vi "ShooterSpeedRegulateV4.1.vi"(8 "Reset PID":bool, 11 "Shooter Speed":T1(ring)) -> (2 "Voltage Output":dbl, 3 "GO GO GO":bool)   [LabVIEW 2012]
uses:
  Robot Global Data.vi
  Max'sToolKit/ConvertVoltageToPercentVbs.vi
panel:
  out "Motor Outputs":cluster{"Error":dbl, dbl, i32}(graph)
  out "Setpoint":dbl
  out "Error (RPS)":dbl
  out "Output":dbl
  out "Speed (RPS)":dbl
  # "Wheel Speed\n0 - DEFAULT/OFF\n1 - close 3pt\n2 - far 3pt\n3 - feeder shot\n4- upside down far 3pt\n\nno more at the moment"
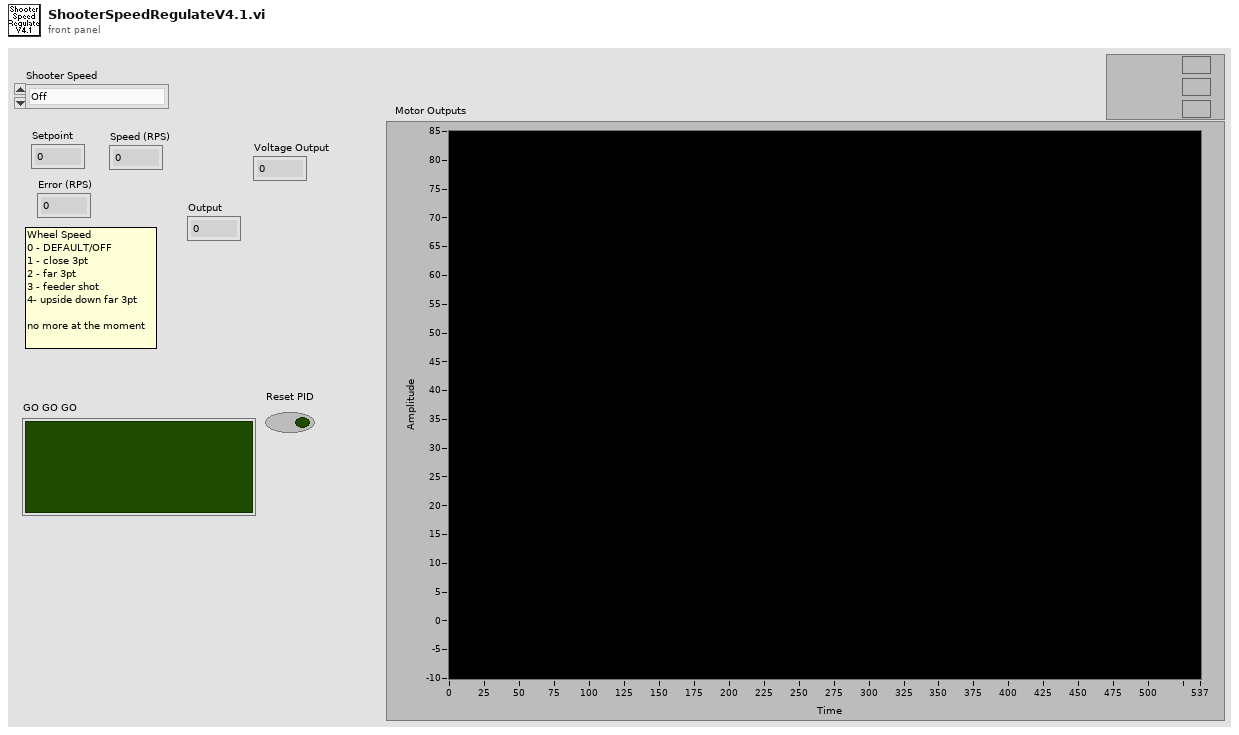
[diagram p1: front panel]
types:
  T1 = enum16{"Off", "Close Pyramid 3pt", "Far Pyramid 3pt", "Feeder Shot", "UD Far 3pt Shot"}
  T2 = cluster{"Target Voltage":dbl, "Target Speed":dbl, "Angle Up?":bool}[]
  T3 = cluster{"Target Voltage":dbl, "Target Speed":dbl, "Angle Up?":bool}
  T4 = typedef "WPI_EncoderDevRef.ctl" = cluster{"DevStatus":errorcluster, "EncoderIndex":T5, "CounterIndex":T6, "DistancePerCount":dbl, "Decoding Type":T7}
  T5 = typedef "FPGA_EncoderIdx.ctl" = enum8{"Enc 0", "Enc 1", "Enc 2", "Enc 3", "Invalid"}
  T6 = typedef "FPGA_CounterCtrSystemIndex.ctl" = enum8{"Ctr 0", "Ctr 1", "Ctr 2", "Ctr 3", "Ctr 4", "Ctr 5", "Ctr 6", "Ctr 7", "Invalid"}
  T7 = typedef "WPI_EncoderType.ctl" = enum16{"1x", "2x", "4x"}
  T8 = cluster{"proportional gain (Kc)":dbl, "integral time (Ti, min)":dbl, "derivative time (Td, min)":dbl}
  T9 = cluster{"Wheel 1 PID-->Out":dbl, "Wheel 1 Out-->PID":dbl}
  T10 = typedef "WPI_MotorControlDeviceRef.ctl" = cluster{"DeviceStatus":errorcluster, "Type":enum16{"PWM", "CAN"}, "PWM":cluster{"Digital Module":T11, "PWM Channel":T12, "DeadBand":T13}, "CAN":cluster{"Device Number":u8, "Control Mode":T14, "Semaphore":T15, "Max Vout":dbl}, "Invert":bool, "TransformRef":T16, "InvTransformRef":T16}
  T11 = typedef "FPGA_TypedefDigitalModule.ctl" = enum16{"Digital Module 1", "Digital Module 2"}
  T12 = typedef "FPGA_DIOPWMChannel.ctl" = enum8{"PWM 1", "PWM 2", "PWM 3", "PWM 4", "PWM 5", "PWM 6", "PWM 7", "PWM 8", "PWM 9", "PWM 10", "Invalid"}
  T13 = typedef "WPI_PWMDeadband.ctl" = cluster{"Name":string, "maxPositivePwm":i32, "minPositivePwm":i32, "centerPwm":i32, "maxNegativePwm":i32, "minNegativePwm":i32, "angularRange":u16}
  T14 = typedef "WPI_CANJaguar_ControlMode.ctl" = enum8{"Percent VBus", "Current", "Speed", "Position", "Voltage"}
  T15 = typedef "Semaphore RefNum" = refnum<k1>
  T16 = typedef "WPI_PWMTransform_ConPane.ctl" = refnum<vi>
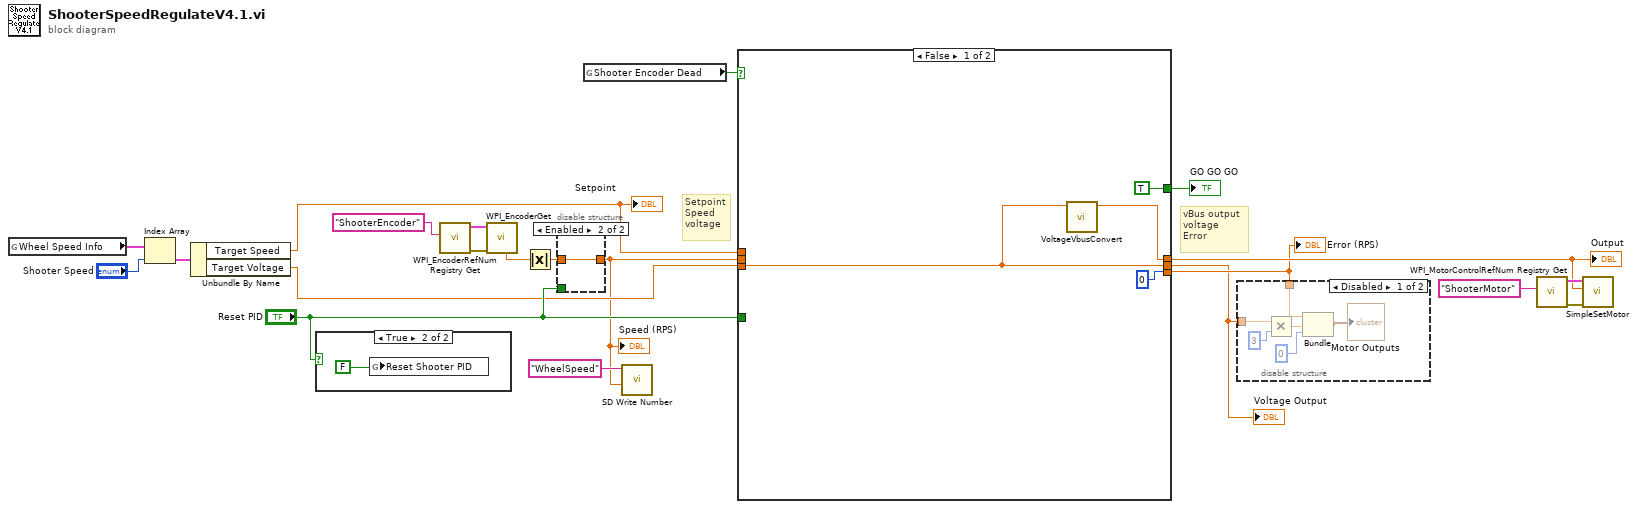
[diagram p0: block diagram]
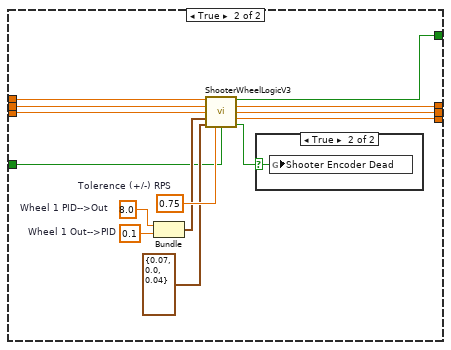
[diagram p2: hidden frame]
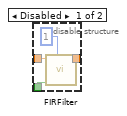
[diagram p5: hidden frame]
diagram:
  # "Setpoint\nSpeed\nvoltage"
  # "vBus output\nvoltage\nError"
  n1 = global read "Robot Global Data.vi" "Wheel Speed Info"() -> (w11:T2)
  n2 = Index Array(array=w11, index="Shooter Speed") -> (element=w10:T3)
  n3 = Unbundle By Name(w10) -> ("Target Speed"=w6:dbl, "Target Voltage"=w9:dbl)
  "Setpoint" <- w6
  n4 = case shown="True" "Reset PID" {
    frame False {
    }
    frame True {
      n5 = global write "Robot Global Data.vi" "Reset Shooter PID"(FALSE) -> ()
    }
  }
  n6 = call <vilib>:"WPI_EncoderRefNum Registry Get.vi"("refnum name"="ShooterEncoder") -> ("error out"=w14:errorcluster, "EncoderDevRef"=w15:T4)  [unwired: 9 in]
  n7 = call <vilib>:"WPI_EncoderGet.vi"("error in (no error)"=w14, "EncoderDevRef"=w15) -> ("Rate"=w13:dbl)  [unwired: 4 in, 5 out]
  n8 = Absolute Value(x=w13) -> (abs(x)=w12:dbl)
  n9 = disable-structure shown="Enabled" {
    disable-tunnel: "Reset PID" -> [w26 _]
    disable-tunnel: w12 -> [w25 w27]
    disable-tunnel: [w24 w27] -> w4
    frame Disabled {
      n10 = call "FIRFilter.vi"("Filter Size"=i8 1, "Reset"=w26, "Input"=w25) -> ("Output"=w24:dbl)  [unwired: 8 in]
    }
    frame Enabled {
    }
  }
  "Speed (RPS)" <- w4
  n11 = global read "Robot Global Data.vi" "Shooter Encoder Dead"() -> (w3:bool)
  n12 = call <vilib>:"SD Write Number.vi"("Numeric"=w4, "Name"="WheelSpeed") -> ()  [unwired: 8 in, 2 out]
  n13 = case shown="False" w3 {
    tunnel: [w30 w44] -> w18
    tunnel: "Reset PID" -> [_ w41]
    tunnel: w9 -> [w29 w38]
    tunnel: [0 w37] -> w8
    tunnel: [w29 w36] -> w7
    tunnel: w6 -> [_ w35]
    tunnel: w4 -> [_ w34]
    tunnel: [TRUE w32] -> w2
    frame False {
      n14 = call-poly "VoltageVbusConvert.vi"("Voltage"=w29) -> ("Vbus"=w30:dbl)  [unwired: 10 in]
    }
    frame True {
      w40 = 0.1  # Wheel 1 Out-->PID
      w39 = 8.0  # Wheel 1 PID-->Out
      w45 = 0.75  # Tolerence (+/-) RPS
      n15 = Bundle("Wheel 1 PID-->Out"=w39, "Wheel 1 Out-->PID"=w40) -> (w43:T9)  [unwired: 1 in]
      n16 = call "ShooterWheelLogicV3.vi"("Setpoint"=w35, "Process Varaible"=w34, "Feedfoward Voltage"=w38, "SwitchZones"=w43, "PID gains"=T8 {"proportional gain (Kc)"=0.07, "integral time (Ti, min)"=0.0, "derivative time (Td, min)"=0.04} ("W1 PID gains"), "Error Margin"=w45, "Reset"=w41) -> ("At Speed"=w32:bool, "Motor Output"=w44:dbl, "Voltage Output"=w36:dbl, "Error"=w37:dbl, "Wheel Died"=w33:bool)  [unwired: 4 in]
      n17 = case shown="True" w33 {
        selector: w33 -> [_ w46]
        frame False {
        }
        frame True {
          n18 = global write "Robot Global Data.vi" "Shooter Encoder Dead"(w46) -> ()
        }
      }
    }
  }
  "Output" <- w18
  "Error (RPS)" <- w8
  "Voltage Output" <- w7
  "GO GO GO" <- w2
  n19 = disable-structure shown="Disabled" {
    disable-tunnel: w8 -> [w51 _]
    disable-tunnel: w7 -> [w47 _]
    frame Disabled {
      n20 = Multiply(x=w47, y=3) -> (x*y=w48:dbl)
      n21 = Bundle("Error"=w51, w48, 0) -> (→"Motor Outputs":cluster{"Error":dbl, dbl, i32})  [unwired: 1 in]
    }
    frame Enabled {
    }
  }
  n22 = call <vilib>:"WPI_MotorControlRefNum Registry Get.vi"("refnum name"="ShooterMotor") -> ("error out"=w19:errorcluster, "MotorControlDevRef"=w20:T10)  [unwired: 9 in]
  n23 = call "SimpleSetMotor.vi"("error in (no error)"=w19, "Output"=w18, "MotorControlDevRef"=w20) -> ()  [unwired: 7 in, 2 out]
